vi "qREC TRACE.vi"(0 "System no.":i32=1 min=1 max=4 step=1, 2 "RecorderIDs to query":string[](array[string]), 3 "TraceIDs to query":i32[](array[numeric]) min=1 max=4 step=1, 5 "error in":errorcluster) -> (14 "List of Recorder Trace Configurations":T1[](array[typedef]) {"ParameterID" min=1 max=4 step=1 format="%x"; "TraceID" min=1 max=4 step=1}, 19 "error out":errorcluster)   [LabVIEW 2020]
doc: "REC? TRACE (Get Data Recorder Trace Configuration)\n\nDescription\nQueries for which variables to be recorded the data recorder traces of the controller are \nconfigured.\n\nFormat\nREC? TRACE[ <RecorderID>[ <TraceID>]]\n\nArguments\nREC? TRACE without arguments queries all data recorders of the controller.\nIf <TraceID> is omitted, all traces for the stated data recorder are queried.\n<RecorderID>\nData recorder, whose configuration is to be queried; to be specified as alias (p. 94) \nThe available data recorders can be queried with USG? SYS (p. 80). \nPossible values: REC_1 to RECn, where n = number of data recorders in the controller\n<TraceID>\nID of the trace to be queried\nThe number of traces of the data recorder can be queried via parameter 0x104. Example:\n>>spv? ram rec_1 - 0x104\n<<RAM REC_1 - 0x104=4\n1 to n, where n = Number of traces of the data recorder\n\nResponse\n{<RecorderID> <TraceID> = <Container Unit> <Function Unit> <ParameterID> LF}\nSee REC TRACE (p. 38) for further details.\n<RecorderStatus>\nCurrent state of the data recorder\nDescriptions of the states can be queried with USG? PROP (p. 79). For further details, see the \nstate diagram for the data recorder (p. 110). \nPossible values: RUN, CFG, WAIT\n\nExample\n>>REC? TRACE\n<<REC_1 1=AXIS_1 - 0x102 \n<<REC_1 2=AXIS_1 TRAJ_1 0x101\n<<REC_1 3=- - - \n<<REC_1 4=- - - \n<<REC_2 1=- - - \n<<REC_2 2=- - - \n<<REC_2 3=- - - \n<<REC_2 4=- - -\n>>REC? TRACE REC_1\n<<REC_1 1=AXIS_1 - 0x102\n<<REC_1 2=AXIS_1 TRAJ_1 0x101\n<<REC_1 3=- - - \n<<REC_1 4=- - -\n>>REC? TRACE REC_1 1\n<<REC_1 1=AXIS_1 - 0x102\n\nNotes\nFor further details, see \"Data Recorder - GCS 3.0\" (p. 107). \n\nUser command level\nUSR"
uses:
  RecorderTraceConfiguration.ctl
panel:
  # "REC? TRACE (Get Data Recorder Trace Configuration)\n\nQueries for which variables to be recorded the data recorder traces of the controller are \nconfigured."
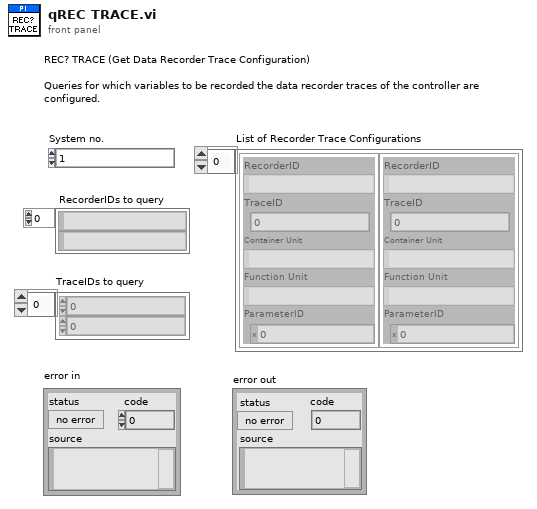
[diagram p1: front panel]
types:
  T1 = typedef "RecorderTraceConfiguration.ctl" = cluster{"RecorderID":string, "TraceID":i32, "Container Unit":string, "Function Unit":string, "ParameterID":i32}
  T2 = typedef "Syntax.ctl" = enum16{"GCS 1.0", "GCS 2.0", "GCS 3.0"}
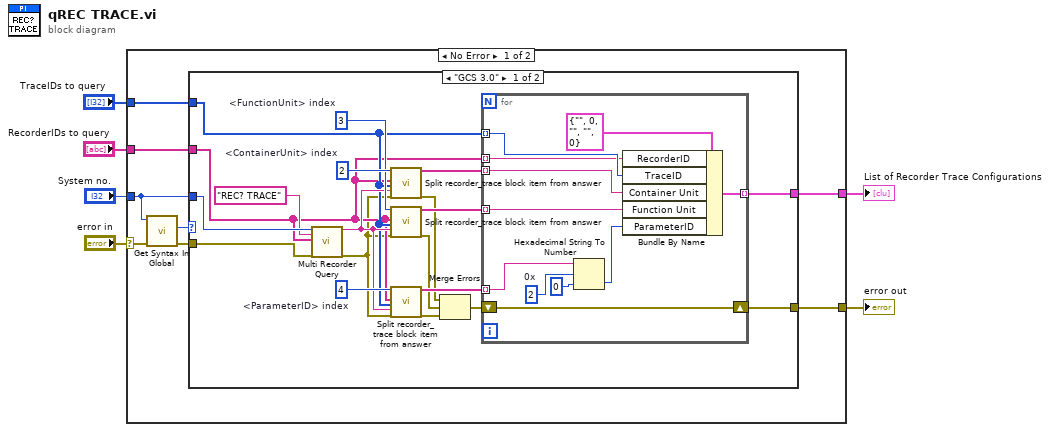
[diagram p0: block diagram]
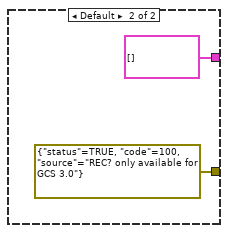
[diagram p2: hidden frame]
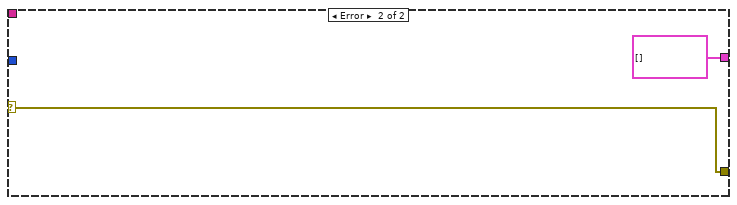
[diagram p3: hidden frame]
diagram:
  n1 = case shown="No Error" "error in" {
    selector: "error in" -> [w14 w48]
    tunnel: [w11 w48] -> w5
    tunnel: "RecorderIDs to query" -> [w9 _]
    tunnel: "System no." -> [w8 _]
    tunnel: [w10 T1[] [] ("List of Recorder Trace Configurations")] -> w1
    tunnel: "TraceIDs to query" -> [w7 _]
    frame No Error {
      n2 = call "Get Syntax In Global.vi"("error in"=w14, "System no."=w8) -> ("error out"=w12:errorcluster, "Syntax"=w13:T2)  [unwired: 8 in]
      n3 = case shown="\"GCS 3.0\"" w13 {
        tunnel: w12 -> [w31 _]
        tunnel: [w29 errorcluster {"status"=TRUE, "code"=100, "source"="REC? only available for GCS 3.0"} ("error out")] -> w11
        tunnel: [w21 T1[] [] ("List of Recorder Trace Configurations")] -> w10
        tunnel: w9 -> [w20 _]
        tunnel: w8 -> [w33 _]
        tunnel: w7 -> [w22 _]
        frame "GCS 3.0" {
          w24 = 4  # <ParameterID> index
          w26 = 3  # <FunctionUnit> index
          w30 = 2  # <ContainerUnit> index
          n4 = call "Multi Recorder Query.vi"("System no."=w33, "Recorder Command"="REC? TRACE" ("format string"), "RecorderIDs to query"=w20, "error in"=w31) -> ("Answer"=w23:string, "error out"=w17:errorcluster)  [unwired: 14 in]
          n5 = call "Split recorder_trace block item from answer.vi"("Slice block item"=w30, "RecorderIDs to query"=w20, "TraceIDs to query"=w22, "Input string"=w23, "error in"=w17) -> ("Sliced text segments"=w28:string[], "error out"=w19:errorcluster)  [unwired: 13 in]
          n6 = call "Split recorder_trace block item from answer.vi"("Slice block item"=w26, "RecorderIDs to query"=w20, "TraceIDs to query"=w22, "Input string"=w23, "error in"=w17) -> ("Sliced text segments"=w27:string[], "error out"=w18:errorcluster)  [unwired: 13 in]
          n7 = call "Split recorder_trace block item from answer.vi"("Slice block item"=w24, "RecorderIDs to query"=w20, "TraceIDs to query"=w22, "Input string"=w23, "error in"=w17) -> ("Sliced text segments"=w25:string[], "error out"=w16:errorcluster)  [unwired: 13 in]
          n8 = Merge Errors(w19, w18, w16) -> (w15:errorcluster)
          n9 = for {
            shift-right: [w44] -> w29
            shift-left: w15 -> [w44]
            tunnel: w28 -> [w41] mode=indexing
            tunnel: w27 -> [w40] mode=indexing
            tunnel: w25 -> [w38] mode=indexing
            tunnel: w22 -> [w43] mode=indexing
            tunnel: [w42] -> w21 mode=indexing
            tunnel: w20 -> [w39] mode=indexing
            w36 = 2  # 0x
            n10 = Hexadecimal String To Number(string=w38, offset=w36, default (0uL)=0 ("ParameterID")) -> (number=w37:i32)  [unwired: 1 out]
            n11 = Bundle By Name(cluster=T1 {"RecorderID"="", "TraceID"=0, "Container Unit"="", "Function Unit"="", "ParameterID"=0} ("RecorderTraceConfiguration"), "RecorderID"=w39, "TraceID"=w43, "Container Unit"=w41, "Function Unit"=w40, "ParameterID"=w37) -> (w42:T1)
          }
        }
        frame Default {
        }
      }
    }
    frame Error {
    }
  }
  "error out" <- w5
  "List of Recorder Trace Configurations" <- w1
